vi "core_wait_for_notification2.vi"(8 "Error in":errorcluster caption="Error in (no error)", 10 "notifier":T1) -> (0 "Error out":errorcluster, 1 "notification":bool, 2 "notifier out":T1)   [LabVIEW 2015]
uses:
  boolean_notifier2.ctl
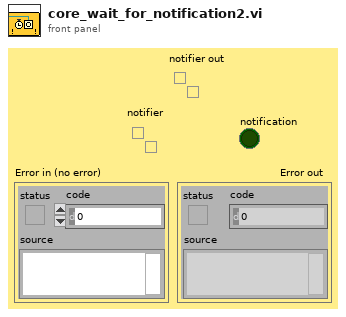
[diagram p1: front panel]
types:
  T1 = typedef "boolean_notifier2.ctl" = refnum<queue>
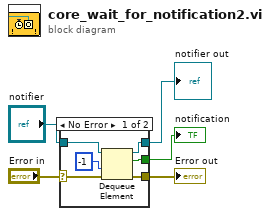
[diagram p0: block diagram]
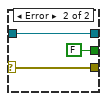
[diagram p2: hidden frame]
diagram:
  n1 = case shown="No Error" "Error in" {
    selector: "Error in" -> [w6 w14]
    tunnel: [w8 w14] -> w4
    tunnel: "notifier" -> [w7 w13]
    tunnel: [w11 w13] -> w2
    tunnel: [w9 FALSE] -> w3
    frame No Error {
      n2 = Dequeue Element(queue=w7, timeout in ms (-1)=-1 ("ms timeout (-1)"), error in (no error)=w6) -> (queue out=w11:T1, element=w9:bool, error out=w8:errorcluster)  [unwired: 1 out]
    }
    frame Error {
    }
  }
  "Error out" <- w4
  "notification" <- w3
  "notifier out" <- w2
